vi "列表框修改.vi"(0 "输入/修改":string[](array[string]), 11 "error in":errorcluster) -> (4 "增加测试信息":string[](array[string]), 15 "error out":errorcluster)   [LabVIEW 2016]
panel:
  out "temp":string[](array[string])
  in  "取消按钮":bool
  in  "确定按钮":bool
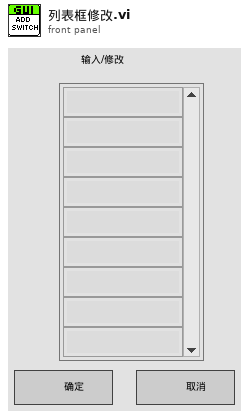
[diagram p1: front panel]
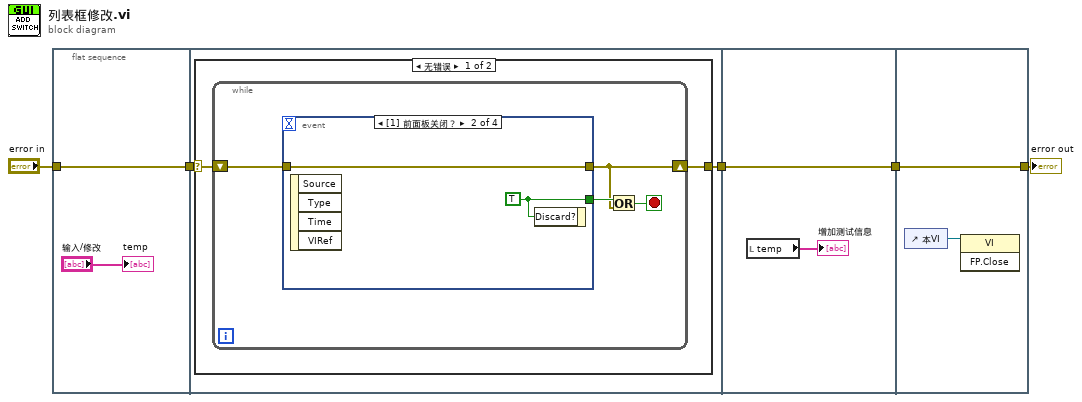
[diagram p0: block diagram]
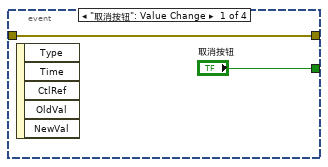
[diagram p2: hidden frame]
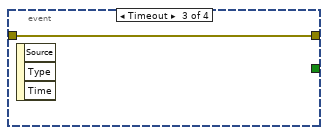
[diagram p3: hidden frame]
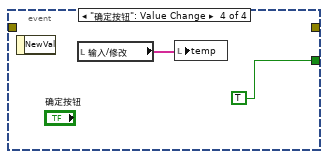
[diagram p4: hidden frame]
diagram:
  n1 = flat-sequence {
    tunnel: "error in" -> [w7]
    tunnel: [w7] -> w3
    tunnel: w3 -> [w8]
    tunnel: [w9] -> w2
    tunnel: w2 -> [w25]
    tunnel: [w25] -> w1
    tunnel: [w27] -> w5
    tunnel: w1 -> [w27]
    frame #0 {
      "temp" <- "输入/修改"
    }
    frame #1 {
      n2 = case shown="无错误" w8 {
        selector: w8 -> [w10 w23]
        tunnel: [w11 w23] -> w9
        frame No Error {
          n3 = while {
            shift-right: [w13] -> w11
            shift-left: w10 -> [w15]
            stop <- w12 stop-if-true
            n4 = event shown="[1] 前面板关闭？" {
              selector: _ -> [_ _ _ _]
              dyn-events: _ -> [_ _ _ _]
              timeout: _ -> [_ _ _ _]
              tunnel: ["取消按钮" w18 _ TRUE ("Discard?")] -> w14
              tunnel: w15 -> [w16 w19 w20 _]
              tunnel: [w16 w19 w20 _] -> w13
              event "取消按钮": Value Change {
                n5 = event-data() -> ()  [unwired: 6 out]
              }
              event Panel Close? {
                w18 = TRUE ("Discard?")
                n6 = event-data() -> ()  [unwired: 5 out]
                n7 = event-data("Discard?"=w18) -> ()  [unwired: 1 in, 1 out]
              }
              event Timeout {
                n8 = event-data() -> ()  [unwired: 4 out]
              }
              event "确定按钮": Value Change {
                n9 = event-data() -> ()  [unwired: 2 out]
                n10 = local read "输入/修改"() -> (w21:string[])
                n11 = local write "temp"(w21) -> ()
              }
            }
            n12 = Or(x=w14, y=w13) -> (x .or. y?=w12:bool)
          }
        }
        frame Error {
        }
      }
    }
    frame #2 {
      n13 = local read "temp"() -> (→"增加测试信息":string[])
    }
    frame #3 {
      n14 = control-ref of="本VI"() -> (w26:refnum<vi>)
      n15 = invoke class="VI" method="FP.Close"(reference=w26) -> ()  [unwired: 2 in, 3 out]
    }
  }
  "error out" <- w5
